vi "Get Dll Path.vi"(7 "Action":enum16{"WriteDllRoot", "GetDllRoot"}(ring), 10 "Root":path) -> (2 "Dll Root Path":path)   [LabVIEW 2019]
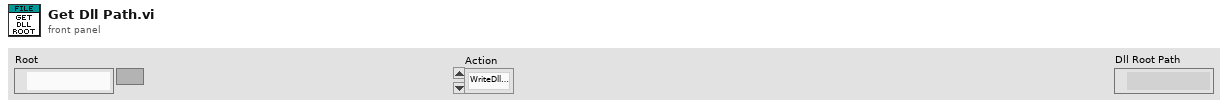
[diagram p1: front panel]
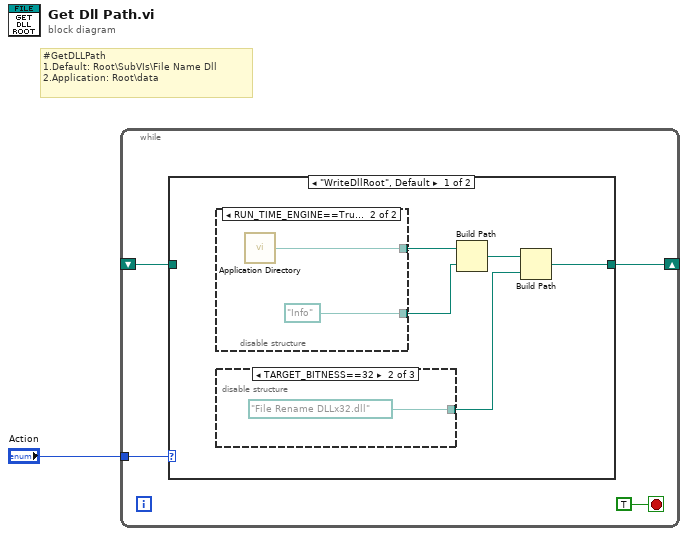
[diagram p0: block diagram]
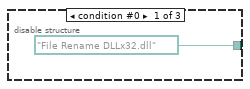
[diagram p2: hidden frame]
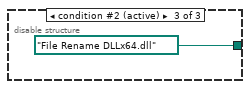
[diagram p3: hidden frame]
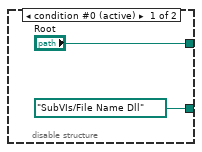
[diagram p4: hidden frame]
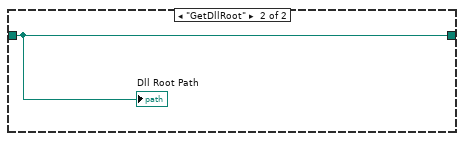
[diagram p5: hidden frame]
diagram:
  # "#GetDLLPath\n1.Default: Root\\SubVIs\\File Name Dll\n2.Application: Root\\data"
  n1 = while {
    shift-right: [w3] -> _
    shift-left: _ -> [w2]
    tunnel: "Action" -> [w4]
    stop <- TRUE stop-if-true
    n2 = case shown="\"WriteDllRoot\", Default" w4 {
      tunnel: [w6 w18] -> w3
      tunnel: w2 -> [_ w18]
      frame "WriteDllRoot", Default {
        n3 = disable-structure shown="RUN_TIME_ENGINE==True" {
          disable-tunnel: [path "SubVIs/File Name Dll" path "Info"] -> w7
          disable-tunnel: ["Root" w16] -> w10
          frame condition #0 (active) {
          }
          frame condition #1 {
            n4 = call <vilib>:"Application Directory.vi"() -> ("Application Directory"=w16:path)
          }
        }
        n5 = disable-structure shown="TARGET_BITNESS==32" {
          disable-tunnel: [path "File Rename DLLx32.dll" path "File Rename DLLx32.dll" path "File Rename DLLx64.dll"] -> w9
          frame condition #0 {
          }
          frame condition #1 {
          }
          frame condition #2 (active) {
          }
        }
        n6 = Build Path(base path=w10, name or relative path=w7) -> (appended path=w8:path)
        n7 = Build Path(base path=w8, name or relative path=w9) -> (appended path=w6:path)
      }
      frame "GetDllRoot" {
        "Dll Root Path" <- w18
      }
    }
  }
